vi "Write T.vi"(8 "error in (no error)":errorcluster, 10 "T":dbl, 11 "PPT Data in":refnum<class "PPT Data.lvclass">) -> (0 "error out":errorcluster, 3 "PPT Data out":refnum<class "PPT Data.lvclass">)   [LabVIEW 2014, in "PPT Library.lvlib" / "PPT Data.lvclass"]
uses:
  PPT Data.lvclass
  PPT Data.lvclass/PPT Data.ctl
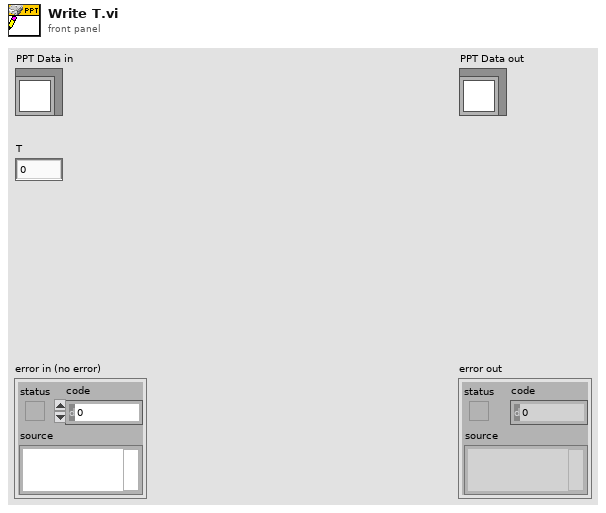
[diagram p1: front panel]
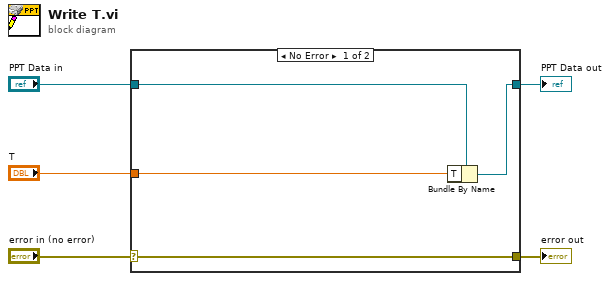
[diagram p0: block diagram]
diagram:
  n1 = case shown="No Error" "error in (no error)" {
    selector: "error in (no error)" -> [w9 w10]
    tunnel: [w9 w10] -> w4
    tunnel: [w7 w11] -> w2
    tunnel: "PPT Data in" -> [w8 w11]
    tunnel: "T" -> [w6 _]
    frame No Error {
      n2 = Bundle By Name(cluster=w8, "T"=w6) -> (w7:refnum<class "PPT Data.lvclass">)
    }
    frame Error {
    }
  }
  "error out" <- w4
  "PPT Data out" <- w2
